vi "COD浓度全局变量.vi"() -> ()   [LabVIEW 2016, in "斯坦道CODMn.lvlib"]
panel:
  in  "COD浓度（mg/L)":dbl
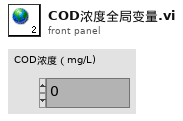
[diagram p1: front panel]
diagram:
